vi "Buffer.Errors.Invalid Buffer.vi"(7 "calling vi name":string, 8 "error in (no error)":errorcluster, 11 "Buffer in":refnum<class "Buffer.lvclass">) -> (0 "error out":errorcluster, 3 "Buffer out":refnum<class "Buffer.lvclass">)   [LabVIEW 2017, in "DSF Core.lvlib" / "Buffer.lvclass"]
uses:
  Buffer.lvclass
  Shared/Constants/DSF.Constants.Library Name.Engine.vi
  <vilib>/NI/Memory Manager/VIs/New Error Cluster Constant (256B).vi
  DSF Core.lvlib
  <vilib>/NI/Memory Manager/Static Error Handling.lvlib
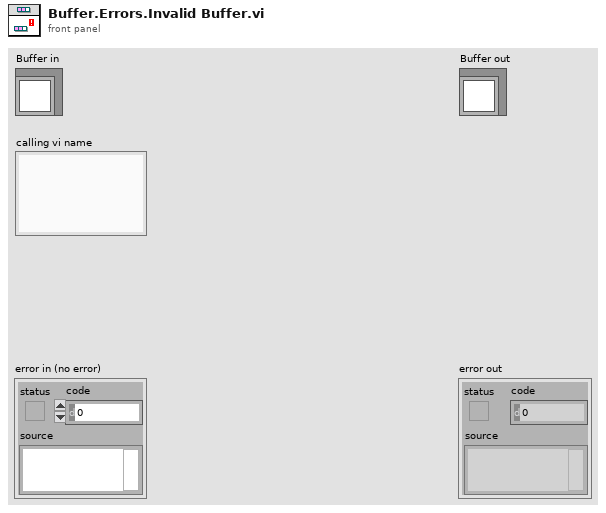
[diagram p1: front panel]
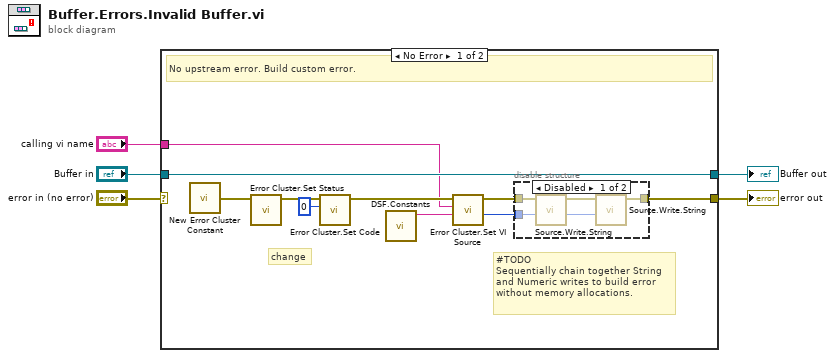
[diagram p0: block diagram]
diagram:
  n1 = case shown="No Error" "error in (no error)" {
    selector: "error in (no error)" -> [_ w22]
    tunnel: "Buffer in" -> [w15 w23]
    tunnel: [w15 w23] -> w4
    tunnel: [w8 w22] -> w3
    tunnel: "calling vi name" -> [w10 _]
    frame No Error {
      # "#TODO\nSequentially chain together String and Numeric writes to build error without memory allocations."
      # "change"
      # "No upstream error. Build custom error."
      n2 = call-poly <vilib>:"New Error Cluster Constant.vi"() -> ("error out"=w6:errorcluster)  [unwired: 1 in]
      n3 = call <vilib>:"Error Cluster.Set Status.vi"("error in"=w6) -> ("error out"=w12:errorcluster)  [unwired: 10 in]
      n4 = call <vilib>:"Error Cluster.Set Code.vi"("code"=0, "error in"=w12) -> ("error out"=w11:errorcluster)  [unwired: 9 in]
      n5 = call-poly "DSF.Constants.vi"() -> ("Engine Library Name"=w14:string)  [unwired: 11 in]
      n6 = call <vilib>:"Error Cluster.Set VI Source.vi"("library name (\"\")"=w14, "vi name"=w10, "error in"=w11) -> ("new offset"=w7:i32, "error out"=w9:errorcluster)  [unwired: 7 in]
      n7 = disable-structure shown="Disabled" {
        disable-tunnel: w9 -> [w20 w21]
        disable-tunnel: [w18 w21] -> w8
        disable-tunnel: w7 -> [w17 _]
        frame Disabled {
          n8 = call <vilib>:"Source.Write.String.vi"("offset"=w17, "error in"=w20) -> ("new offset"=w16:i32, "error out"=w19:errorcluster)  [unwired: 8 in]
          n9 = call <vilib>:"Source.Write.String.vi"("offset"=w16, "error in"=w19) -> ("error out"=w18:errorcluster)  [unwired: 8 in, 1 out]
        }
        frame Enabled {
        }
      }
    }
    frame Error {
      # "Upstream error. Pass through."
    }
  }
  "error out" <- w3
  "Buffer out" <- w4
